vi "Camera Shutter_Luan2024.05.01.vi"(8 "error in (no error)":errorcluster, 10 "Exposure Time":dbl, 11 "Refnum in":T1="Cam Extra (3)") -> (0 "error out":errorcluster, 3 "Refnum out":T1="Cam Extra (3)")   [LabVIEW 2023]
uses:
  <vilib>/userDefined/High Color/IMAQdx.ctl
  <resource>/objmgr/imaqdx.rc
panel:
  out "Exposure Time (Out)":dbl
  # "ExposureMode"
  # "ExposureAuto"
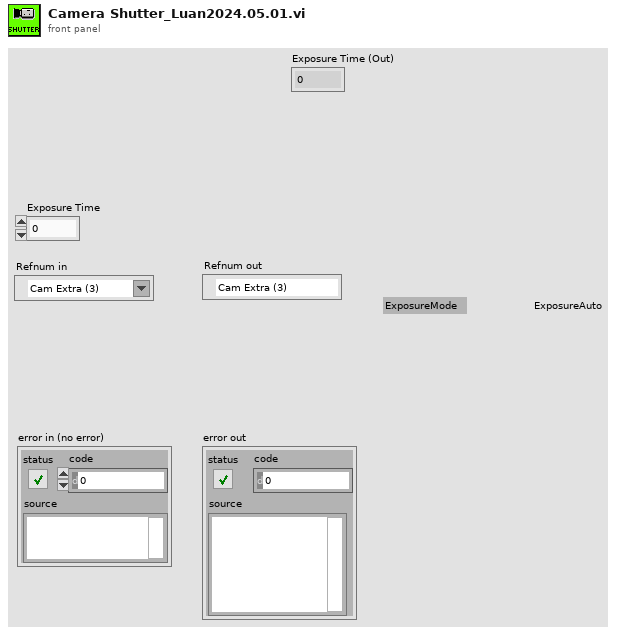
[diagram p1: front panel]
types:
  T1 = typedef "IMAQdx.ctl" = refnum<k21>
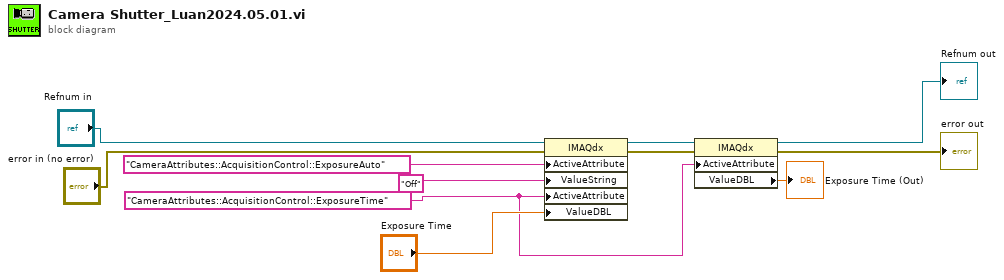
[diagram p0: block diagram]
diagram:
  w2 = "CameraAttributes::AcquisitionControl::ExposureTime" ("ActiveAttribute")
  n1 = property class="IMAQdx"(reference="Refnum in", error in="error in (no error)", "ActiveAttribute"="CameraAttributes::AcquisitionControl::ExposureAuto", "ValueString"="Off", "ActiveAttribute"=w2, "ValueDBL"="Exposure Time") -> (reference out=w4:T1, error out=w6:errorcluster)
  n2 = property class="IMAQdx"(reference=w4, error in=w6, "ActiveAttribute"=w2) -> (reference out=→"Refnum out":T1, error out=→"error out":errorcluster, "ValueDBL"=→"Exposure Time (Out)":dbl)
